vi "Obtain Frame Buffer.vi"(7 "Buffer Size (10k)":i32=10000 format="%.0p", 8 "error in":errorcluster, 10 "Create (F)":bool) -> (0 "error out":errorcluster, 3 "queue out":refnum<queue>)   [LabVIEW 2025, in "CAN-LIN Raw Bus Capture.lvclass"]
uses:
  CAN-LIN Raw Bus Capture.lvclass
  <vilib>/xnet/xnet.llb/XNET Frame CAN.ctl
  <vilib>/xnet/xnet.llb/XNET Frame Type CAN.ctl
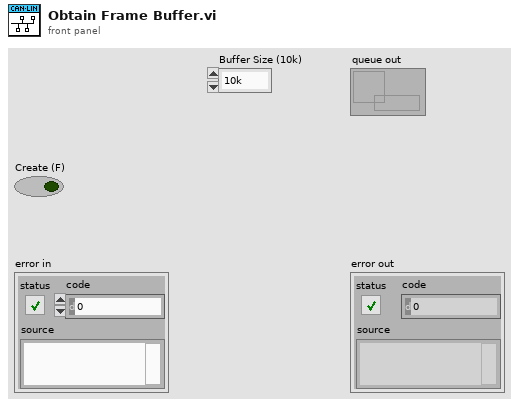
[diagram p1: front panel]
types:
  T1 = typedef "XNET Frame CAN.ctl" = cluster{"timestamp":timestamp, "payload":u8[], "identifier":u32, "type":T2, "extended?":bool, "echo?":bool}
  T2 = typedef "XNET Frame Type CAN.ctl" = u8
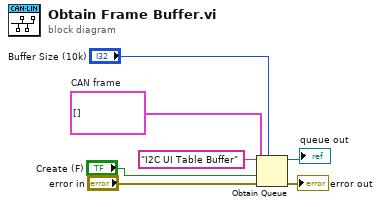
[diagram p0: block diagram]
diagram:
  w2 = T1[] []  # CAN frame
  n1 = Obtain Queue(max queue size (-1, unlimited)="Buffer Size (10k)", name (unnamed)="I2C UI Table Buffer", element data type=w2, create if not found? (T)="Create (F)", error in (no error)="error in") -> (queue out=→"queue out":refnum<queue>, error out=→"error out":errorcluster)  [unwired: 1 out]
